vi "Test Deserialize Enum.vi"(8 "error in (no error)":errorcluster) -> (0 "error out":errorcluster)   [LabVIEW 2013]
uses:
  src/Deserializer/JSON Deserializer/JSON Deserializer.lvclass
  <vilib>/addons/_JKI Toolkits/Caraya/classes/Test/Test.lvclass
  <vilib>/addons/_JKI Toolkits/Caraya/classes/Assert/Assert.lvclass
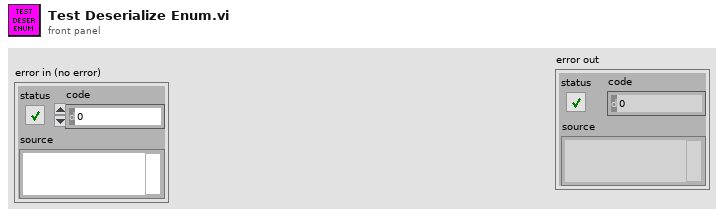
[diagram p1: front panel]
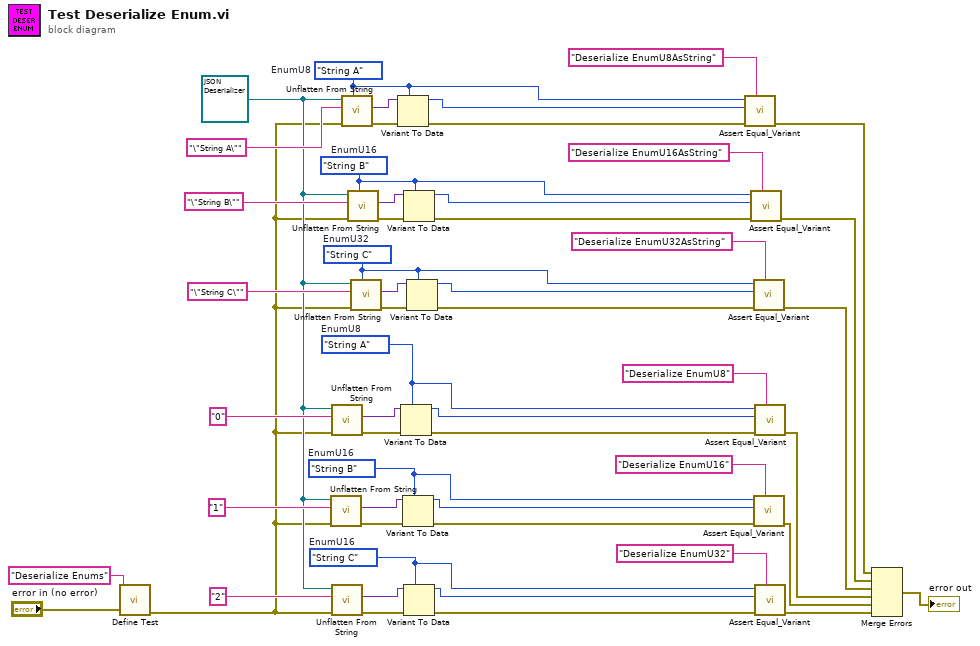
[diagram p0: block diagram]
diagram:
  w9 = enum32{"String A", "String B", "String C"}."String C"  # EnumU32
  w20 = enum16{"String A", "String B", "String C"}."String B"  # EnumU16
  w28 = enum16{"String A", "String B", "String C"}."String B"  # EnumU16
  w29 = enum32{"String A", "String B", "String C"}."String C"  # EnumU16
  w1 = enum8{"String A", "String B", "String C"}."String A"  # EnumU8
  w2 = enum8{"String A", "String B", "String C"}."String A"  # EnumU8
  w4 = refnum<class "JSON Deserializer.lvclass"> refnum ("JKI JSON Serialization.lvlib:JSON Deserializer.lvclass")
  n1 = call <vilib>:"Define Test.vi"("error in (no error)"="error in (no error)", "Label (VI Title)"="Deserialize Enums") -> ("error out"=w3:errorcluster)  [unwired: 9 in]
  n2 = call-dynamic "Unflatten From String.vi"("error in (no error)"=w3, "String"="1", "Deserializer in"=w4) -> ("error out"=w22:errorcluster, "Variant"=w25:variant)  [unwired: 6 in, 1 out]
  n3 = call-dynamic "Unflatten From String.vi"("error in (no error)"=w3, "String"="0", "Deserializer in"=w4) -> ("error out"=w39:errorcluster, "Variant"=w35:variant)  [unwired: 6 in, 1 out]
  n4 = call-dynamic "Unflatten From String.vi"("error in (no error)"=w3, "String"="2", "Deserializer in"=w4) -> ("error out"=w41:errorcluster, "Variant"=w33:variant)  [unwired: 6 in, 1 out]
  n5 = call-dynamic "Unflatten From String.vi"("Type and Defaults"=w2, "error in (no error)"=w3, "String"="\"String A\"", "Deserializer in"=w4) -> ("error out"=w45:errorcluster, "Variant"=w46:variant)  [unwired: 5 in, 1 out]
  n6 = call-dynamic "Unflatten From String.vi"("Type and Defaults"=w20, "error in (no error)"=w3, "String"="\"String B\"", "Deserializer in"=w4) -> ("error out"=w16:errorcluster, "Variant"=w15:variant)  [unwired: 5 in, 1 out]
  n7 = call-dynamic "Unflatten From String.vi"("Type and Defaults"=w9, "error in (no error)"=w3, "String"="\"String C\"", "Deserializer in"=w4) -> ("error out"=w13:errorcluster, "Variant"=w14:variant)  [unwired: 5 in, 1 out]
  n8 = Variant To Data(error in=w45, type=w2, Variant=w46) -> (data=w42:enum8{"String A", "String B", "String C"}, error out=w43:errorcluster)
  n9 = Variant To Data(error in=w39, type=w1, Variant=w35) -> (data=w30:enum8{"String A", "String B", "String C"}, error out=w36:errorcluster)
  n10 = Variant To Data(error in=w22, type=w28, Variant=w25) -> (data=w27:enum16{"String A", "String B", "String C"}, error out=w24:errorcluster)
  n11 = Variant To Data(error in=w16, type=w20, Variant=w15) -> (data=w19:enum16{"String A", "String B", "String C"}, error out=w18:errorcluster)
  n12 = Variant To Data(error in=w41, type=w29, Variant=w33) -> (data=w31:enum32{"String A", "String B", "String C"}, error out=w34:errorcluster)
  n13 = Variant To Data(error in=w13, type=w9, Variant=w14) -> (data=w10:enum32{"String A", "String B", "String C"}, error out=w11:errorcluster)
  n14 = call <vilib>:"Assert Equal_Variant.vi"("Label"="Deserialize EnumU8AsString", "error in (no error)"=w43, "Y"=w42, "X"=w2) -> ("error out"=w21:errorcluster)  [unwired: 7 in]
  n15 = call <vilib>:"Assert Equal_Variant.vi"("Label"="Deserialize EnumU16AsString", "error in (no error)"=w18, "Y"=w19, "X"=w20) -> ("error out"=w8:errorcluster)  [unwired: 7 in]
  n16 = call <vilib>:"Assert Equal_Variant.vi"("Label"="Deserialize EnumU32AsString", "error in (no error)"=w11, "Y"=w10, "X"=w9) -> ("error out"=w7:errorcluster)  [unwired: 7 in]
  n17 = call <vilib>:"Assert Equal_Variant.vi"("Label"="Deserialize EnumU16", "error in (no error)"=w24, "Y"=w27, "X"=w28) -> ("error out"=w48:errorcluster)  [unwired: 7 in]
  n18 = call <vilib>:"Assert Equal_Variant.vi"("Label"="Deserialize EnumU8", "error in (no error)"=w36, "Y"=w30, "X"=w1) -> ("error out"=w50:errorcluster)  [unwired: 7 in]
  n19 = call <vilib>:"Assert Equal_Variant.vi"("Label"="Deserialize EnumU32", "error in (no error)"=w34, "Y"=w31, "X"=w29) -> ("error out"=w51:errorcluster)  [unwired: 7 in]
  n20 = Merge Errors(w21, w8, w7, w50, w48, w51) -> (→"error out":errorcluster)
